vi "StartControlVIs.vi"(8 "entrée d'erreur (pas d'erreur)":errorcluster, 10 "This VI":refnum<vi>, 11 "Control in":refnum<class "Control-Server.lvclass">) -> (0 "sortie d'erreur":errorcluster, 3 "Control out":refnum<class "Control-Server.lvclass">)   [LabVIEW 2018, in "Control-Server.lvclass"]
uses:
  Classes/Control/Control-Server/Control-Server.lvclass
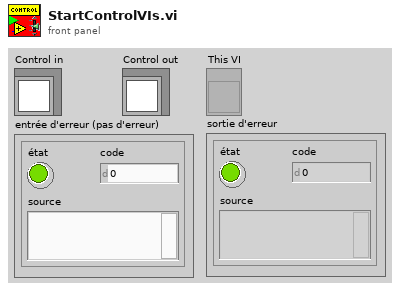
[diagram p1: front panel]
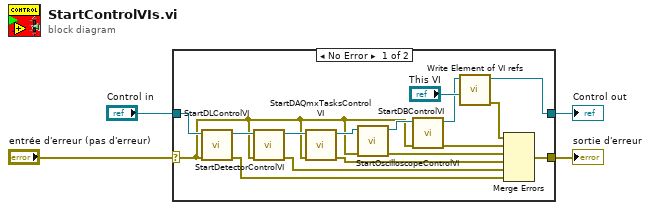
[diagram p0: block diagram]
diagram:
  n1 = case shown="No Error" "entrée d'erreur (pas d'erreur)" {
    selector: "entrée d'erreur (pas d'erreur)" -> [w5 w22]
    tunnel: [w15 w21] -> w4
    tunnel: "Control in" -> [w20 w21]
    tunnel: [w18 w22] -> w3
    frame No Error {
      n2 = call "StartDLControlVI.vi"("entrée d'erreur (pas d'erreur)"=w5, "Control en entrée"=w20) -> ("sortie d'erreur"=w19:errorcluster, "Control en sortie"=w17:refnum<class "Control-Server.lvclass">)  [unwired: 8 in]
      n3 = call "StartDetectorControlVI.vi"("entrée d'erreur (pas d'erreur)"=w5, "Control en entrée"=w17) -> ("sortie d'erreur"=w12:errorcluster, "Control en sortie"=w14:refnum<class "Control-Server.lvclass">)  [unwired: 8 in]
      n4 = call "StartDAQmxTasksControlVI.vi"("entrée d'erreur (pas d'erreur)"=w5, "Control en entrée"=w14) -> ("sortie d'erreur"=w13:errorcluster, "Control en sortie"=w10:refnum<class "Control-Server.lvclass">)  [unwired: 8 in]
      n5 = call "StartOscilloscopeControlVI.vi"("entrée d'erreur (pas d'erreur)"=w5, "Control en entrée"=w10) -> ("sortie d'erreur"=w11:errorcluster, "Control en sortie"=w9:refnum<class "Control-Server.lvclass">)  [unwired: 8 in]
      n6 = call "StartDBControlVI.vi"("entrée d'erreur (pas d'erreur)"=w5, "Control en entrée"=w9) -> ("sortie d'erreur"=w6:errorcluster, "Control en sortie"=w8:refnum<class "Control-Server.lvclass">)  [unwired: 8 in]
      n7 = call "Write Element of VI refs.vi"("vi reference"="This VI", "Control in"=w8) -> ("error out"=w7:errorcluster, "Control out"=w15:refnum<class "Control-Server.lvclass">)  [unwired: 8 in]
      n8 = Merge Errors(w7, w6, w11, w13, w12, w19) -> (w18:errorcluster)
    }
    frame Error {
    }
  }
  "Control out" <- w4
  "sortie d'erreur" <- w3
